vi "ECG.vi"() -> ()   [LabVIEW 2018]
panel:
  in  "Ascendido":bool
  out "Waveform Chart":dynamicdata(graph)
  in  "PC/ECG":bool
  # "Electrocardiograma"
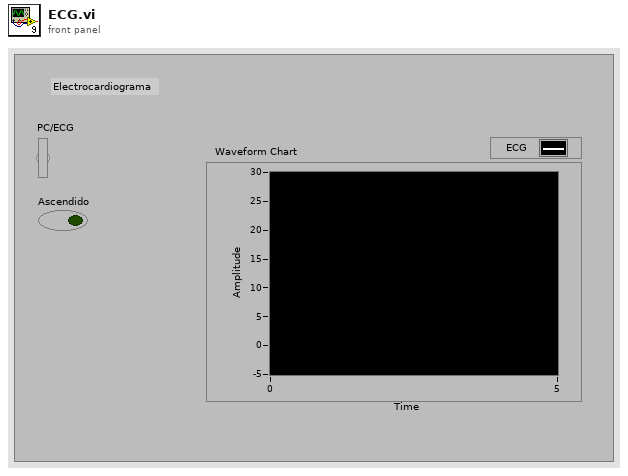
[diagram p1: front panel]
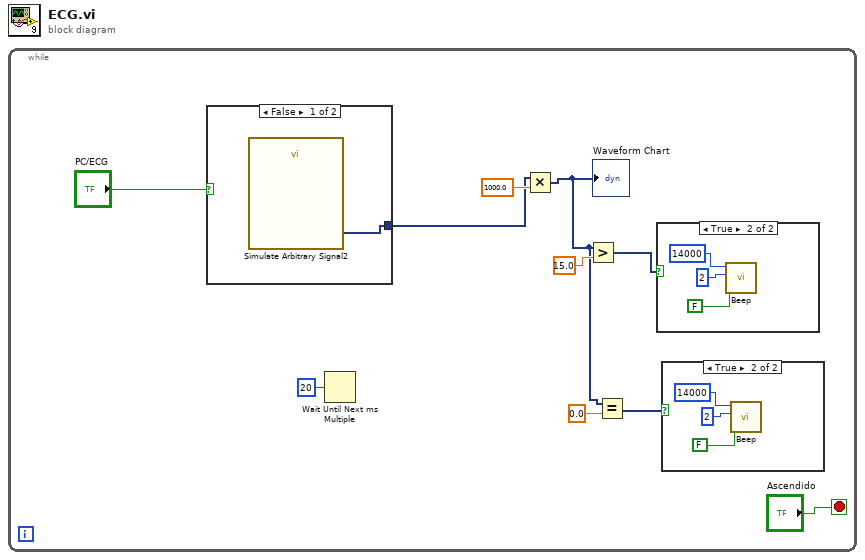
[diagram p0: block diagram]
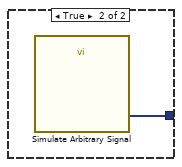
[diagram p4: hidden frame]
diagram:
  n1 = while {
    stop <- "Ascendido" stop-if-true
    n2 = case shown="False" "PC/ECG" {
      tunnel: [w17 w18] -> w8
      frame False {
        n3 = call "Simulate Arbitrary Signal2"() -> ("Signal"=w17:dynamicdata)  [unwired: 9 in, 2 out]
      }
      frame True {
        n4 = call "Simulate Arbitrary Signal"() -> ("Signal"=w18:dynamicdata)  [unwired: 9 in, 2 out]
      }
    }
    n5 = Wait Until Next ms Multiple(millisecond multiple=u32 20) -> ()  [unwired: 1 out]
    n6 = Multiply(x=w8, y=1000.0) -> (x*y=w3:dynamicdata)
    "Waveform Chart" <- w3
    n7 = Greater?(x=w3, y=15.0) -> (0:w6:dynamicdata)
    n8 = Equal?(x=w3, y=0.0) -> (x = y?=w5:dynamicdata)
    n9 = case shown="True" w6 {
      frame False {
      }
      frame True {
        n10 = call <vilib>:"Beep.vi"("use system alert? (T)"=FALSE, "duration (msec)"=u32 2, "frequency (Hz)"=u32 14000) -> ()  [unwired: 9 in]
      }
    }
    n11 = case shown="True" w5 {
      frame False {
      }
      frame True {
        n12 = call <vilib>:"Beep.vi"("use system alert? (T)"=FALSE, "duration (msec)"=u32 2, "frequency (Hz)"=u32 14000) -> ()  [unwired: 9 in]
      }
    }
  }
